vi "GraphLimit01.vi"(6 "Numeric 2":dbl, 9 "Numeric":dbl, 10 "Array in":dbl[](array[numeric]), 11 "Array 3":dbl[](array[numeric])) -> (3 "Array out":dbl[](array[numeric]))   [LabVIEW 2024]
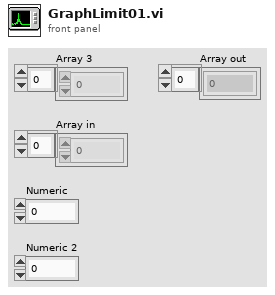
[diagram p1: front panel]
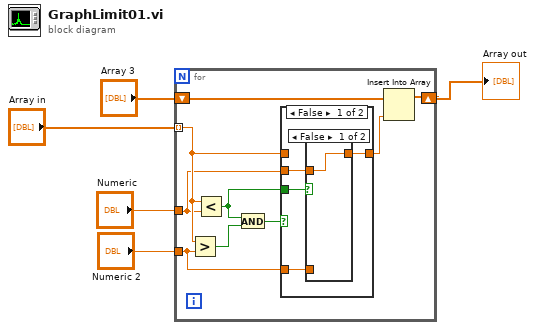
[diagram p0: block diagram]
diagram:
  n1 = for {
    shift-right: [w12] -> w2
    shift-left: "Array 3" -> [w13]
    tunnel: "Numeric" -> [w6]
    tunnel: "Numeric 2" -> [w7]
    tunnel: "Array in" -> [w9] mode=indexing
    n2 = Greater?(x=w9, y=w7) -> (0:w11:bool)
    n3 = Less?(x=w9, y=w6) -> (x < y?=w8:bool)
    n4 = And(x=w8, y=w11) -> (x .and. y?=w14:bool)
    n5 = case shown="False" w14 {
      tunnel: w9 -> [_ w21]
      tunnel: w6 -> [w15 _]
      tunnel: w7 -> [w17 _]
      tunnel: w8 -> [w18 _]
      tunnel: [w16 w21] -> w10
      frame False {
        n6 = case shown="False" w18 {
          tunnel: w17 -> [_ w20]
          tunnel: [w19 w20] -> w16
          tunnel: w15 -> [w19 _]
          frame False {
          }
          frame True {
          }
        }
      }
      frame True {
      }
    }
    n7 = Insert Into Array(array=w13, new element=w10) -> (w12:dbl[])  [unwired: 1 in]
  }
  "Array out" <- w2
